vi "resultsColumnsStats.vi"(6 "Indicies to Output":bool[](array[boolean]), 8 "Analysis Info cluster":T1[](array[typedef]) {"Sync Delay Time (s)" format="%.4f"; "Total Meas Time (s)" format="%_5g"; "Sd Error in Variance" format="%_3g"; "Skew_u" format="%_3g"; "% u'/U" format="%_3g"; "Sd Error in Mean" format="%_3g"; "Kurt_u" format="%_3g"; "u^4" format="%_3g"; "u^3" format="%_3g"; "U" format="%_3g"; "u^2" format="%_3g"}, 10 "chValuesIn":string[](array[string]), 11 "chNamesIn":string[](array[string])) -> (2 "chValuesOut":string[](array[string]), 3 "chNamesOut":string[](array[string]), 5 "dupsArray":i32[](array[numeric]))   [LabVIEW 2022 SP3]
uses:
  Controls/Analysis_info_cluster.ctl
  Controls/Inst_type.ctl
  Controls/Instrument_Array.ctl
  Controls/channelState.ctl
  Globals/Meas_global.vi
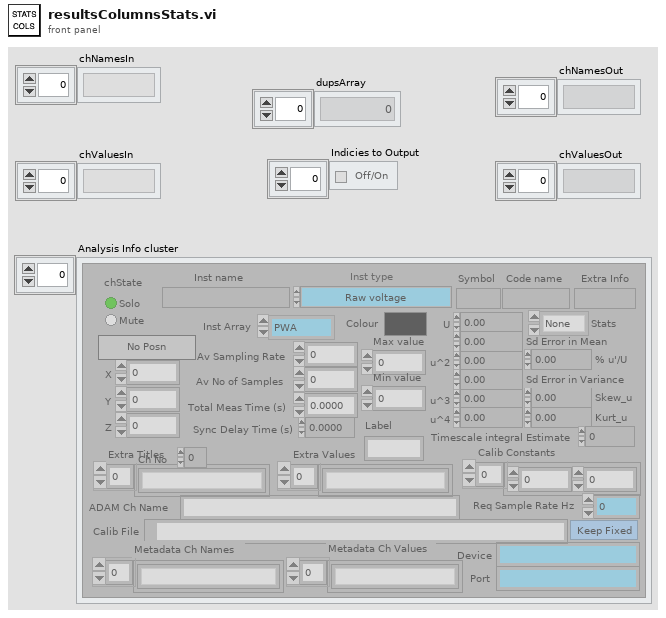
[diagram p1: front panel]
types:
  T1 = typedef "Analysis_info_cluster.ctl" = cluster{"Colour":u32, "Inst type":T2, "Inst name":string, "Symbol":string, "Code name":string, "Extra Info":string, "Inst Array":T3, "Extra Titles":string[], "Extra Values":string[], "U":dbl, "u^2":dbl, "u^3":dbl, "u^4":dbl, "Skew_u":dbl, "Kurt_u":dbl, "Sd Error in Mean":dbl, "% u'/U":dbl, "X":dbl, "Y":dbl, "Z":dbl, "Timescale integral Estimate":dbl, "Sd Error in Variance":dbl, "Calib File":path, "Calib Constants":dbl[], "Output Position":bool, "Stats":enum16{"None", "Basic", "Full"}, "Av Sampling Rate":dbl, "Av No of Samples":dbl, "Total Meas Time (s)":dbl, "ADAM Ch Name":string, "Max value":dbl, "Min value":dbl, "Req Sample Rate Hz":dbl, "Sync Delay Time (s)":dbl, "Ch No":i16, "Device":string, "Use Latest Calib":bool, "Port":string, "Metadata Ch Names":string[], "Metadata Ch Values":string[], "Label":string, "chState":T4}
  T2 = typedef "Inst_type.ctl" = enum16{"Raw voltage", "Raw with zero offsetting", "Propeller anemometer", "Pressure Transducer", "Pitot-static tube", "Hot wire", "Cross wire 1", "Cross wire 2", "Generic Linear", "Generic Polynomial", "Generic BackPoly", "Fast FID", "Thermocouple", "Cold wire", "Pulsed Wire", "LDA Vel", "LDA Tran time", "LDA Arr time", "Microphone"}
  T3 = typedef "Instrument_Array.ctl" = enum16{"PWA", "LDA", "Analogue"}
  T4 = typedef "channelState.ctl" = enum32{"No Selection", "Solo", "Mute"}
  T5 = typedef "XY_Plot_Cluster.ctl" = cluster{"First Name":string, "Second Name":string, "X axis name":string, "Y axis name":string, "X array":dbl[], "Y array":dbl[], "Weighting":dbl[]}
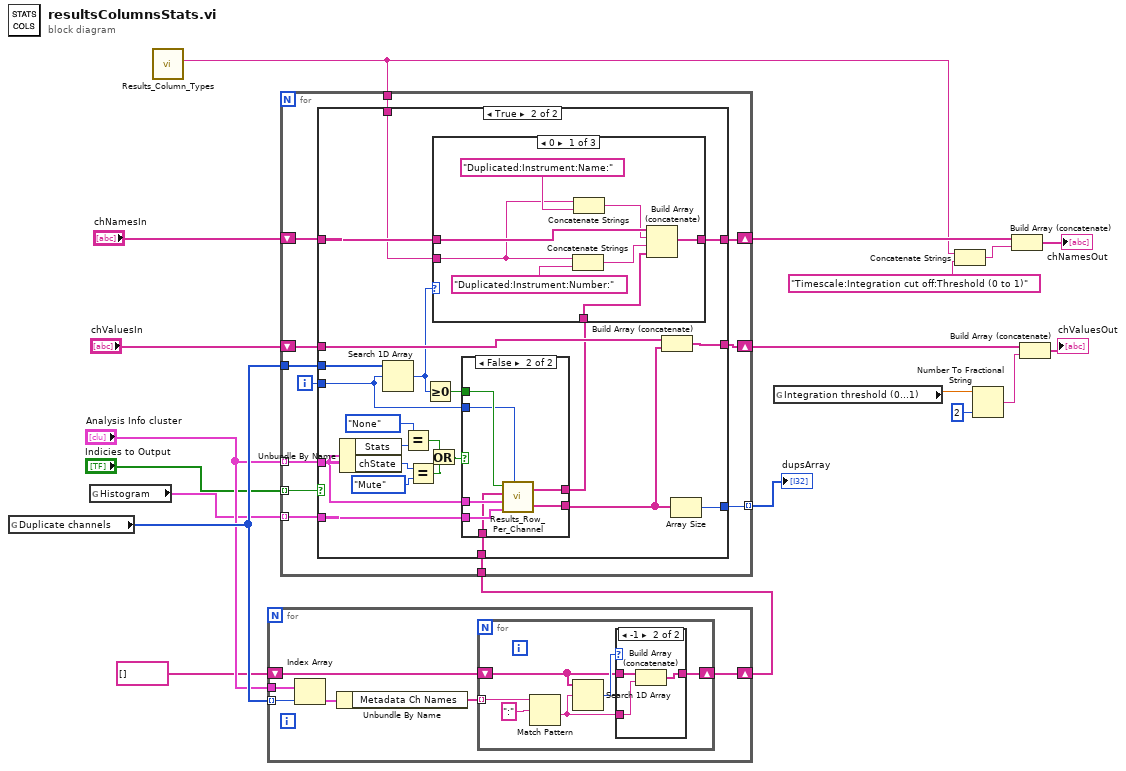
[diagram p0: block diagram]
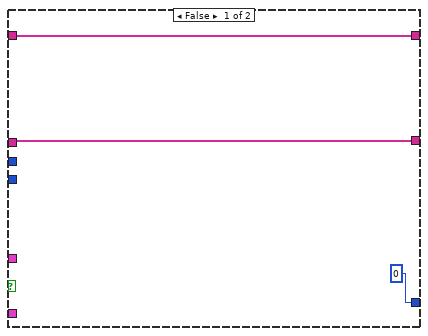
[diagram p3: hidden frame]
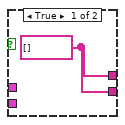
[diagram p4: hidden frame]
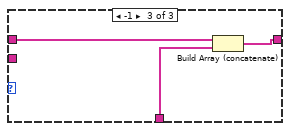
[diagram p6: hidden frame]
diagram:
  n1 = global read "Meas_global.vi" "Duplicate channels"() -> (w19:i32[])
  n2 = global read "Meas_global.vi" "Histogram"() -> (w14:T5[])
  n3 = call "Results_Column_Types.vi"() -> ("Metadata"=w1:string)  [unwired: 9 in, 2 out]
  n4 = for {
    tunnel: "Analysis Info cluster" -> [w25]
    tunnel: w19 -> [w24] mode=indexing
    shift-right: [w20] -> w16
    shift-left: string[] [] -> [w21]
    n5 = Index Array(array=w25, index=w24) -> (element=w23:T1)
    n6 = Unbundle By Name(w23) -> ("Metadata Ch Names"=w22:string[])
    n7 = for {
      tunnel: w22 -> [w31] mode=indexing
      shift-right: [w27] -> w20
      shift-left: w21 -> [w28]
      n8 = Match Pattern(string=w31, regular expression=":") -> (after substring=w26:string)  [unwired: 1 in, 3 out]
      n9 = Search 1D Array(1D array=w28, element=w26) -> (index of element=w29:i32)  [unwired: 1 in]
      n10 = case shown="-1" w29 {
        tunnel: w26 -> [_ w35]
        tunnel: w28 -> [w32 w34]
        tunnel: [w32 w33] -> w27
        frame Default {
        }
        frame -1 {
          n11 = Build Array (concatenate)(w34, w35) -> (w33:string[])
        }
      }
    }
  }
  n12 = for {
    shift-right: [w44] -> w10
    shift-left: "chNamesIn" -> [w46]
    shift-right: [w47] -> w12
    shift-left: "chValuesIn" -> [w45]
    tunnel: "Analysis Info cluster" -> [w39] mode=indexing
    tunnel: [w43] -> w13 mode=indexing
    tunnel: w19 -> [w41]
    tunnel: w14 -> [w40] mode=indexing
    tunnel: w16 -> [w38]
    tunnel: "Indicies to Output" -> [w37] mode=indexing
    tunnel: w1 -> [w36]
    i -> [w42]
    n13 = case shown="True" w37 {
      tunnel: [w49 w72] -> w47
      tunnel: w46 -> [w50 w71]
      tunnel: w45 -> [w49 w70]
      tunnel: [w50 w69] -> w44
      tunnel: [0 w68] -> w43
      tunnel: w42 -> [_ w60]
      tunnel: w41 -> [_ w67]
      tunnel: w40 -> [_ w66]
      tunnel: w39 -> [_ w65]
      tunnel: w38 -> [_ w62]
      tunnel: w36 -> [_ w51]
      frame False {
      }
      frame True {
        n14 = Unbundle By Name(w65) -> ("Stats"=w58:enum16{"None", "Basic", "Full"}, "chState"=w56:T4)
        n15 = Search 1D Array(1D array=w67, element=w60) -> (index of element=w64:i32)  [unwired: 1 out]
        n16 = Equal?(x=enum16{"None", "Basic", "Full"}."None" ("Stats"), y=w58) -> (x = y?=w54:bool)
        n17 = Equal?(x=w56, y=channelState."Mute" ("chState")) -> (x = y?=w53:bool)
        n18 = Greater Or Equal To 0?(x=w64) -> (x >= 0?=w63:bool)
        n19 = Or(x=w54, y=w53) -> (x .or. y?=w52:bool)
        n20 = case shown="False" w52 {
          tunnel: [w73 w80] -> w61
          tunnel: [w73 w79] -> w59
          tunnel: w66 -> [_ w78]
          tunnel: w65 -> [_ w77]
          tunnel: w63 -> [_ w76]
          tunnel: w62 -> [_ w75]
          tunnel: w60 -> [_ w74]
          frame True {
            w73 = string[] [] ("Channel Names")
          }
          frame False {
            n21 = call "Results_Row_Per_Channel.vi"("Duplicate Channel"=w76, "Duplicate Metadata channels"=w75, "Analysis_info_cluster"=w77, "Histogram Info"=w78, "Index"=w74) -> ("Channel Names"=w80:string[], "Channel Values"=w79:string[])
          }
        }
        n22 = case shown="0" w64 {
          tunnel: w71 -> [w88 w89 w92]
          tunnel: [w86 w89 w91] -> w69
          tunnel: w61 -> [w87 _ w90]
          tunnel: w51 -> [w82 _ _]
          frame 0 {
            n23 = Concatenate Strings(w82, "Duplicated:Instrument:Number:") -> (w84:string)
            n24 = Concatenate Strings(w82, "Duplicated:Instrument:Name:") -> (w81:string)
            n25 = Build Array (concatenate)(w88, w81, w84, w87) -> (w86:string[])
          }
          frame 1, Default {
          }
          frame -1 {
            n26 = Build Array (concatenate)(w92, w90) -> (w91:string[])
          }
        }
        n27 = Build Array (concatenate)(w70, w59) -> (w72:string[])
        n28 = Array Size(array=w59) -> (size(s)=w68:i32)
      }
    }
  }
  "dupsArray" <- w13
  n29 = global read "Meas_global.vi" "Integration threshold (0...1)"() -> (w7:dbl)
  n30 = Concatenate Strings(w1, "Timescale:Integration cut off:Threshold (0 to 1)") -> (w2:string)
  n31 = Number To Fractional String(number=w7, precision (6)=i16 2) -> (F-format string=w4:string)  [unwired: 2 in]
  n32 = Build Array (concatenate)(w10, w2) -> (→"chNamesOut":string[])
  n33 = Build Array (concatenate)(w12, w4) -> (→"chValuesOut":string[])
